vi "Cannon Finish.vi"   [LabVIEW 2013]
types:
  T1 = typedef "WPI_SolenoidDevRef.ctl" = cluster{"DevStatus":errorcluster, "Solenoid Module":T2, "Forward Solenoid Channel":T3, "Reverse Solenoid Channel":T3}
  T2 = typedef "FPGA_TypedefSolenoidModule.ctl" = enum16{"Solenoid Module 1", "Solenoid Module 2"}
  T3 = typedef "WPI_SolenoidChannel.ctl" = enum8{"Solenoid 1", "Solenoid 2", "Solenoid 3", "Solenoid 4", "Solenoid 5", "Solenoid 6", "Solenoid 7", "Solenoid 8", "Invalid"}
  T4 = typedef "WPI_MotorControlDeviceRef.ctl" = cluster{"DeviceStatus":errorcluster, "Type":enum16{"PWM", "CAN"}, "PWM":cluster{"Digital Module":T5, "PWM Channel":T6, "DeadBand":T7}, "CAN":cluster{"Device Number":u8, "Control Mode":T8, "Semaphore":T9, "Max Vout":dbl}, "Invert":bool, "TransformRef":T10, "InvTransformRef":T10}
  T5 = typedef "FPGA_TypedefDigitalModule.ctl" = enum16{"Digital Module 1", "Digital Module 2"}
  T6 = typedef "FPGA_DIOPWMChannel.ctl" = enum8{"PWM 1", "PWM 2", "PWM 3", "PWM 4", "PWM 5", "PWM 6", "PWM 7", "PWM 8", "PWM 9", "PWM 10", "Invalid"}
  T7 = typedef "WPI_PWMDeadband.ctl" = cluster{"Name":string, "maxPositivePwm":i32, "minPositivePwm":i32, "centerPwm":i32, "maxNegativePwm":i32, "minNegativePwm":i32, "angularRange":u16}
  T8 = typedef "WPI_CANJaguar_ControlMode.ctl" = enum8{"Percent VBus", "Current", "Speed", "Position", "Voltage"}
  T9 = typedef "Semaphore RefNum" = refnum<k1>
  T10 = typedef "WPI_PWMTransform_ConPane.ctl" = refnum<vi>
  T11 = typedef "WPI_DigitalInputDevRef.ctl" = cluster{"DevStatus":errorcluster, "DIO Channel":T12, "Digital Module":T5}
  T12 = typedef "FPGA_DIOChannel.ctl" = enum8{"DIO 1", "DIO 2", "DIO 3", "DIO 4", "DIO 5", "DIO 6", "DIO 7", "DIO 8", "DIO 9", "DIO 10", "DIO 11", "DIO 12", "DIO 13", "DIO 14", "Invalid"}
  T13 = typedef "WPI_GyroDevRef.ctl" = cluster{"DevStatus":errorcluster, "Analog Module":T14, "Analog Channel":T15, "Offset":dbl, "Gain (VoltsPerDegree/Second)":dbl}
  T14 = typedef "FPGA_TypedefAnalogModule.ctl" = enum16{"Analog Module 1", "Analog Module 2"}
  T15 = typedef "FPGA_AIChannel.ctl" = enum8{"AI 1", "AI 2", "AI 3", "AI 4", "AI 5", "AI 6", "AI 7", "AI 8", "Invalid"}
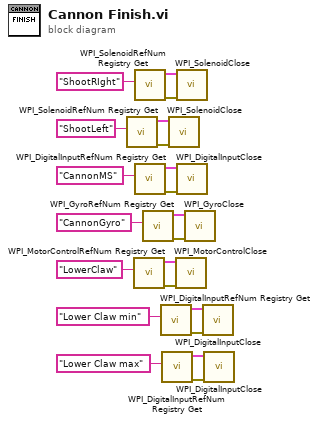
[diagram p0: block diagram]
diagram:
  n1 = call <vilib>:"WPI_SolenoidRefNum Registry Get.vi"("refnum name"="ShootLeft") -> ("error out"=w16:errorcluster, "SolenoidDevRef"=w15:T1)  [unwired: 9 in]
  n2 = call <vilib>:"WPI_MotorControlRefNum Registry Get.vi"("refnum name"="LowerClaw") -> ("error out"=w9:errorcluster, "MotorControlDevRef"=w8:T4)  [unwired: 9 in]
  n3 = call <vilib>:"WPI_SolenoidRefNum Registry Get.vi"("refnum name"="ShootRIght") -> ("error out"=w18:errorcluster, "SolenoidDevRef"=w17:T1)  [unwired: 9 in]
  n4 = call <vilib>:"WPI_DigitalInputRefNum Registry Get.vi"("refnum name"="CannonMS") -> ("error out"=w14:errorcluster, "DigitalInputDevRef"=w13:T11)  [unwired: 9 in]
  n5 = call <vilib>:"WPI_GyroRefNum Registry Get.vi"("refnum name"="CannonGyro") -> ("error out"=w11:errorcluster, "GyroDevRef"=w12:T13)  [unwired: 9 in]
  n6 = call <vilib>:"WPI_DigitalInputRefNum Registry Get.vi"("refnum name"="Lower Claw min") -> ("error out"=w3:errorcluster, "DigitalInputDevRef"=w4:T11)  [unwired: 9 in]
  n7 = call <vilib>:"WPI_DigitalInputRefNum Registry Get.vi"("refnum name"="Lower Claw max") -> ("error out"=w2:errorcluster, "DigitalInputDevRef"=w1:T11)  [unwired: 9 in]
  n8 = call <vilib>:"WPI_SolenoidClose.vi"("error in (no error)"=w16, "SolenoidDevRef"=w15) -> ()  [unwired: 9 in, 1 out]
  n9 = call <vilib>:"WPI_MotorControlClose.vi"("error in (no error)"=w9, "MotorControlDevRef"=w8) -> ()  [unwired: 9 in, 1 out]
  n10 = call <vilib>:"WPI_SolenoidClose.vi"("error in (no error)"=w18, "SolenoidDevRef"=w17) -> ()  [unwired: 9 in, 1 out]
  n11 = call <vilib>:"WPI_DigitalInputClose.vi"("error in (no error)"=w14, "DigitalInputDevRef"=w13) -> ()  [unwired: 9 in, 1 out]
  n12 = call <vilib>:"WPI_GyroClose.vi"("error in (no error)"=w11, "GyroDevRef"=w12) -> ()  [unwired: 9 in, 1 out]
  n13 = call <vilib>:"WPI_DigitalInputClose.vi"("error in (no error)"=w3, "DigitalInputDevRef"=w4) -> ()  [unwired: 9 in, 1 out]
  n14 = call <vilib>:"WPI_DigitalInputClose.vi"("error in (no error)"=w2, "DigitalInputDevRef"=w1) -> ()  [unwired: 9 in, 1 out]
